vi "Configure Voltage.vi"(7 "Voltage Integration Time (10: 10)":dbl(ring)=10.0 items=["0.02"=0.02, "0.2"=0.2, "1"=1.0, "10"=10.0, "100"=100.0], 8 "error in (no error)":errorcluster, 9 "Auto Impedance (F: Disable)":bool, 10 "Voltage Bandwidth (20: 20 Hz)":i32(ring)=20 items=["3"=3, "20"=20, "200"=200], 11 "VISA resource name":refnum<visa-resource-name>) -> (0 "error out":errorcluster, 3 "VISA resource name out":refnum<visa-resource-name>)   [LabVIEW 2013, in "Agilent 3446X Series.lvlib"]
doc: "Configures the settings for voltage measurements.\n\n<b>Note(s) : </b>\nFor EDU34450A model, Only Auto Impedance is supported."
uses:
  <instrlib>/Agilent 3446X Series/Agilent 3446X Series.lvlib
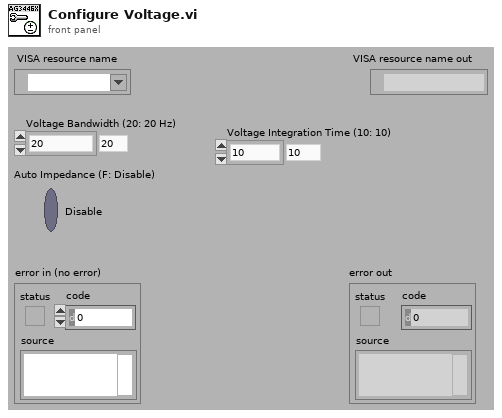
[diagram p1: front panel]
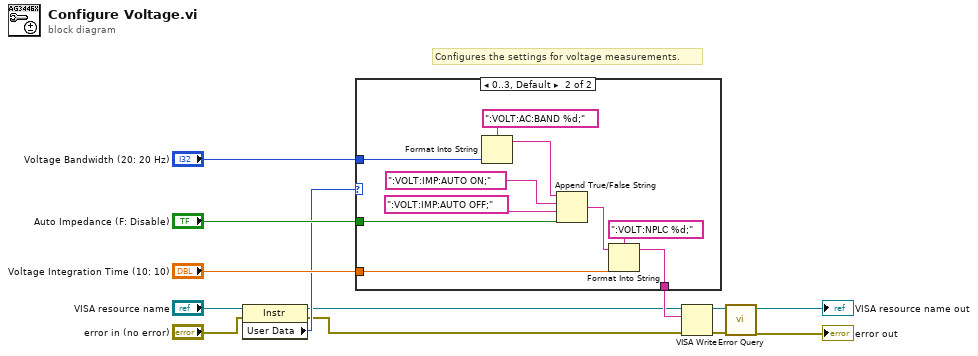
[diagram p0: block diagram]
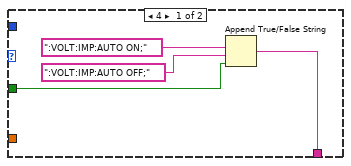
[diagram p2: hidden frame]
diagram:
  # "Configures the settings for voltage measurements."
  n1 = property class="Instr"(reference="VISA resource name", error in="error in (no error)") -> (reference out=w3:refnum<visa-resource-name>, error out=w1:errorcluster, "User Data"=w4:u32)
  n2 = case shown="0..3, Default" w4 {
    tunnel: "Voltage Bandwidth (20: 20 Hz)" -> [_ w26]
    tunnel: "Auto Impedance (F: Disable)" -> [w14 w19]
    tunnel: "Voltage Integration Time (10: 10)" -> [_ w21]
    tunnel: [w15 w20] -> w6
    frame 4 {
      n3 = Append True/False String(1:w14, 2:":VOLT:IMP:AUTO OFF;", 3:":VOLT:IMP:AUTO ON;") -> (0:w15:string)  [unwired: 1 in]
    }
    frame 0..3, Default {
      n4 = Format Into String(format string=":VOLT:AC:BAND %d;", w26) -> (resulting string=w25:string)  [unwired: 2 in, 1 out]
      n5 = Append True/False String(1:w19, 2:":VOLT:IMP:AUTO OFF;", 3:":VOLT:IMP:AUTO ON;", 4:w25) -> (0:w18:string)
      n6 = Format Into String(format string=":VOLT:NPLC %d;", initial string=w18, w21) -> (resulting string=w20:string)  [unwired: 1 in, 1 out]
    }
  }
  n7 = VISA Write(VISA resource name=w3, write buffer=w6, error in (no error)=w1) -> (VISA resource name out=w11:refnum<visa-resource-name>, error out=w10:errorcluster)  [unwired: 1 out]
  n8 = call <instrlib>:"Error Query.vi"("error in (no error)"=w10, "VISA resource name"=w11) -> ("error out"=→"error out":errorcluster, "VISA resource name out"=→"VISA resource name out":refnum<visa-resource-name>)  [unwired: 8 out]
